vi "TestWriteMultipleImages.vi"() -> ()   [LabVIEW 2018]
uses:
  LVTiffWriter.lvlib
panel:
  in  "Compress?":bool=TRUE
  out "Image":T1(plugin-control)
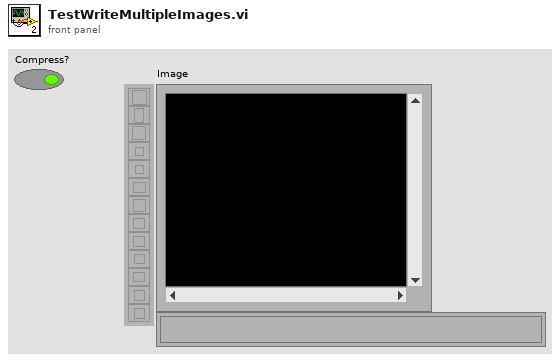
[diagram p1: front panel]
types:
  T1 = typedef "IMAQ Image.ctl" = refnum<image>
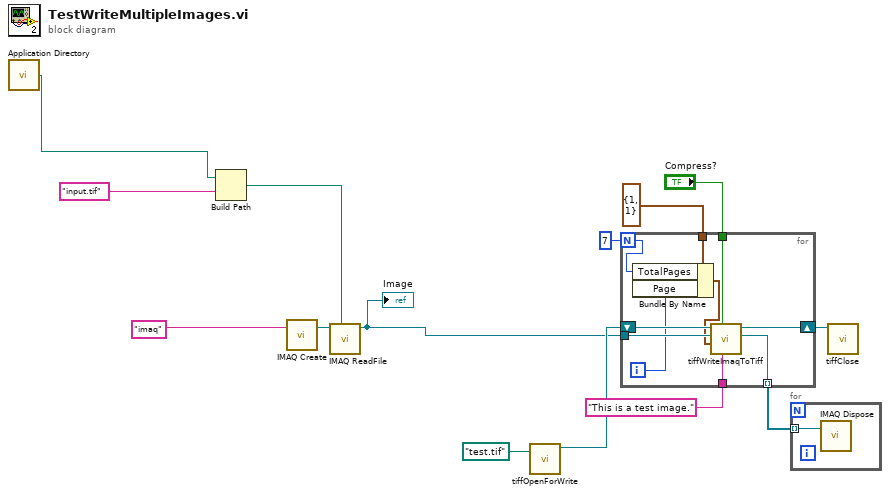
[diagram p0: block diagram]
diagram:
  n1 = call <vilib>:"Application Directory.vi"() -> ("Application Directory"=w1:path)
  n2 = Build Path(base path=w1, name or relative path="input.tif" ("File Path")) -> (appended path=w5:path)
  n3 = call "IMAQ Create"("Image Name"="imaq" ("initial string")) -> ("New Image"=w4:T1)  [unwired: 4 in, 1 out]
  n4 = call "IMAQ ReadFile"("File Path"=w5, "Image"=w4) -> ("Image Out"=w10:T1)  [unwired: 5 in, 4 out]
  "Image" <- w10
  n5 = call "tiffOpenForWrite.vi"("Path"=path "test.tif") -> ("TiffOut"=w11:refnum<k24>)  [unwired: 10 in]
  n6 = for {
    N: 7 -> [w19]
    tunnel: "Compress?" -> [w23]
    tunnel: w10 -> [w21]
    shift-right: [w24] -> w14
    shift-left: w11 -> [w22]
    tunnel: cluster{"Page":i32, "TotalPages":i32} {"Page"=1, "TotalPages"=1} ("Multipage") -> [w20]
    tunnel: [w16] -> w8 mode=indexing
    tunnel: "This is a test image." ("ImageDescription") -> [w15]
    i -> [w18]
    n7 = Bundle By Name(cluster=w20, "TotalPages"=w19, "Page"=w18) -> (w17:cluster{"Page":i32, "TotalPages":i32})
    n8 = call "tiffWriteImaqToTiff.vi"("ImageDescription"=w15, "Compress?"=w23, "Multipage"=w17, "ImaqIn"=w21, "TiffIn"=w22) -> ("ImaqOut"=w16:T1, "TiffOut"=w24:refnum<k24>)  [unwired: 5 in]
  }
  n9 = for {
    tunnel: w8 -> [w25] mode=indexing
    n10 = call "IMAQ Dispose"("Image"=w25) -> ()  [unwired: 5 in, 1 out]
  }
  n11 = call "tiffClose.vi"("Tiff in"=w14) -> ()  [unwired: 10 in, 1 out]
